vi "decodeImageString.vi"(8 "error in (no error)":errorcluster, 10 "encodedImage":string, 11 "ImageAnalyser in":refnum<class "ImageAnalyser.lvclass">) -> (0 "error out":errorcluster, 1 "isImage?":bool, 2 "ImageData":T1, 3 "ImageAnalyser out":refnum<class "ImageAnalyser.lvclass">)   [LabVIEW 2009, in "Tools.lvlib" / "Imaging.lvlib" / "ImageAnalyser.lvclass"]
uses:
  ImageAnalyser.lvclass
  <vilib>/xml/Close Reference(Node).vi
  <vilib>/xml/Load XML String.vi
  <vilib>/xml/NI_XML.lvlib
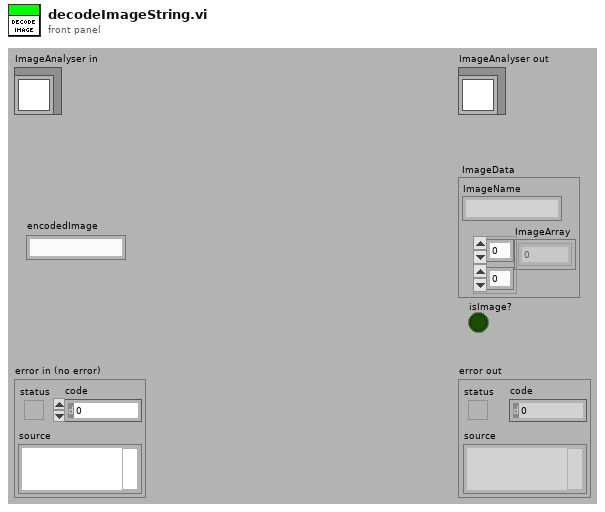
[diagram p1: front panel]
types:
  T1 = cluster{"ImageName":string, "ImageArray":sgl[][]}
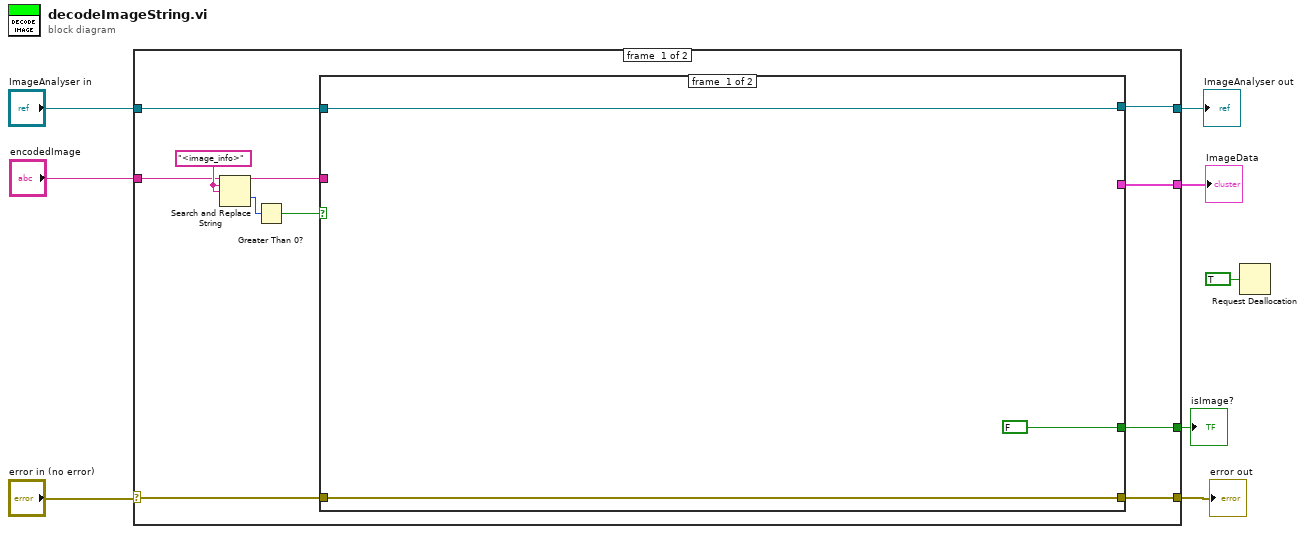
[diagram p0: block diagram]
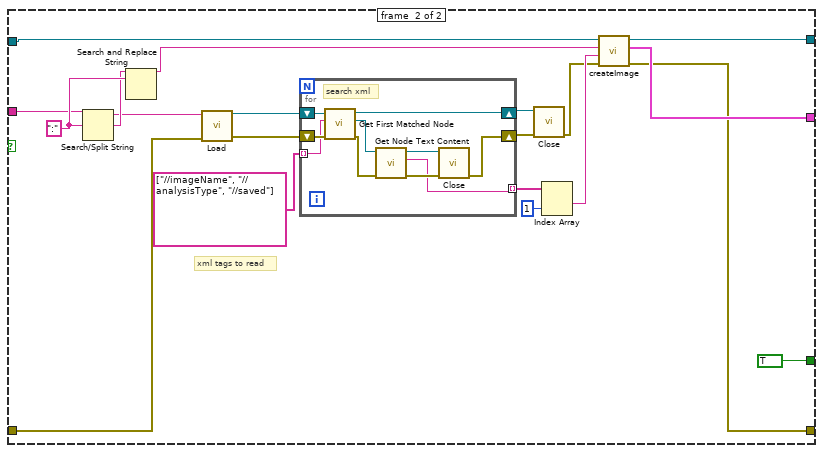
[diagram p2: hidden frame]
diagram:
  n1 = case shown="No Error" "error in (no error)" {
    selector: "error in (no error)" -> [w14 w54]
    tunnel: [w11 w54] -> w7
    tunnel: [w12 w53] -> w5
    tunnel: "ImageAnalyser in" -> [w15 w53]
    tunnel: "encodedImage" -> [w17 _]
    tunnel: [w10 _] -> w3
    tunnel: [w9 _] -> w2
    frame #0 {
      w19 = "<image_info>"
      n2 = Search and Replace String(input string=w17, search string=w19, replace string=w19) -> (result string=w13:string, offset past replacement=w18:i32)  [unwired: 5 in, 2 out]
      n3 = Greater Than 0?(x=w18) -> (x > 0?=w16:bool)
      n4 = case shown="True" w16 {
        tunnel: w15 -> [w22 w33]
        tunnel: w14 -> [w21 w38]
        tunnel: w13 -> [_ w40]
        tunnel: [w22 w24] -> w12
        tunnel: [w21 w23] -> w11
        tunnel: [_ w26] -> w10
        tunnel: [FALSE TRUE] -> w9
        frame #0 {
        }
        frame #1 {
          w42 = ":"
          # "xml tags to read"
          n5 = Search/Split String(string=w40, search string/char (-)=w42) -> (substring before match=w39:string, match + rest of string=w41:string)  [unwired: 1 in, 1 out]
          n6 = Search and Replace String(input string=w41, search string=w42) -> (result string=w31:string)  [unwired: 6 in, 3 out]
          n7 = call-poly <vilib>:"Load.vi"("XML string"=w39, "error in (no error)"=w38) -> ("DOM document out"=w37:refnum<k20>, "error out"=w36:errorcluster)  [unwired: 11 in, 1 out]
          n8 = for {
            shift-right: [w44] -> w29
            shift-left: w37 -> [w48]
            shift-right: [w45] -> w28
            shift-left: w36 -> [w47]
            tunnel: string[] ["//imageName", "//analysisType", "//saved"] -> [w46] mode=indexing
            tunnel: [w43] -> w34 mode=indexing
            # "search xml"
            n9 = call <vilib>:"Get First Matched Node.vi"("error in (no error)"=w47, "XPath expression"=w46, "node in"=w48) -> ("error out"=w52:errorcluster, "node result"=w51:refnum<k20>, "node out"=w44:refnum<k20>)  [unwired: 6 in]
            n10 = call <vilib>:"Get Node Text Content.vi"("error in (no error)"=w52, "node in"=w51) -> ("error out"=w50:errorcluster, "node text"=w43:string, "node out"=w49:refnum<k20>)  [unwired: 7 in]
            n11 = call-poly <vilib>:"Close.vi"("error in (no error)"=w50, "node"=w49) -> ("error out"=w45:errorcluster)  [unwired: 7 in]
          }
          n12 = call-poly <vilib>:"Close.vi"("error in (no error)"=w28, "node"=w29) -> ("error out"=w27:errorcluster)  [unwired: 7 in]
          n13 = Index Array(array=w34, index #2=1) -> (element #1=w30:string)  [unwired: 1 in, 1 out]
          n14 = call "createImage.vi"("error in (no error)"=w27, "ImageName"=w30, "imageString"=w31, "ImageAnalyser in"=w33) -> ("error out"=w23:errorcluster, "ImageData"=w26:T1, "ImageAnalyser out"=w24:refnum<class "ImageAnalyser.lvclass">)  [unwired: 5 in]
        }
      }
    }
    frame #1 {
    }
  }
  "error out" <- w7
  "ImageAnalyser out" <- w5
  "ImageData" <- w3
  "isImage?" <- w2
  n15 = Request Deallocation(TRUE ("flag")) -> ()
